vi "ReversedEngineering GetClassAttributes.vi"(1 "Path(CtrlRenum used if Path is empty)":path, 2 "CtlRefnum":refnum<vi>, 5 "error in (no error)":errorcluster) -> (12 "LibraryName":string, 15 "attributeInfo":T1[](array[typedef]), 19 "error out":errorcluster)   [LabVIEW 2020]
uses:
  <resource>/Framework/Providers/Open_GDS/UML/UmlEditor_class/UmlEditor.lvclass
  <resource>/Framework/Providers/Open_GDS/ClassProviders/Common/CommonVIs/CommonVIs_AttributeInfoType.ctl
  <resource>/Framework/Providers/Open_GDS/ClassProviders/Common/CommonVIs/CommonVIs_VisibilityType.ctl
  <resource>/Framework/Providers/Open_GDS/ClassProviders/Common/CommonVIs/CommonVIs_AttributeDataType.ctl
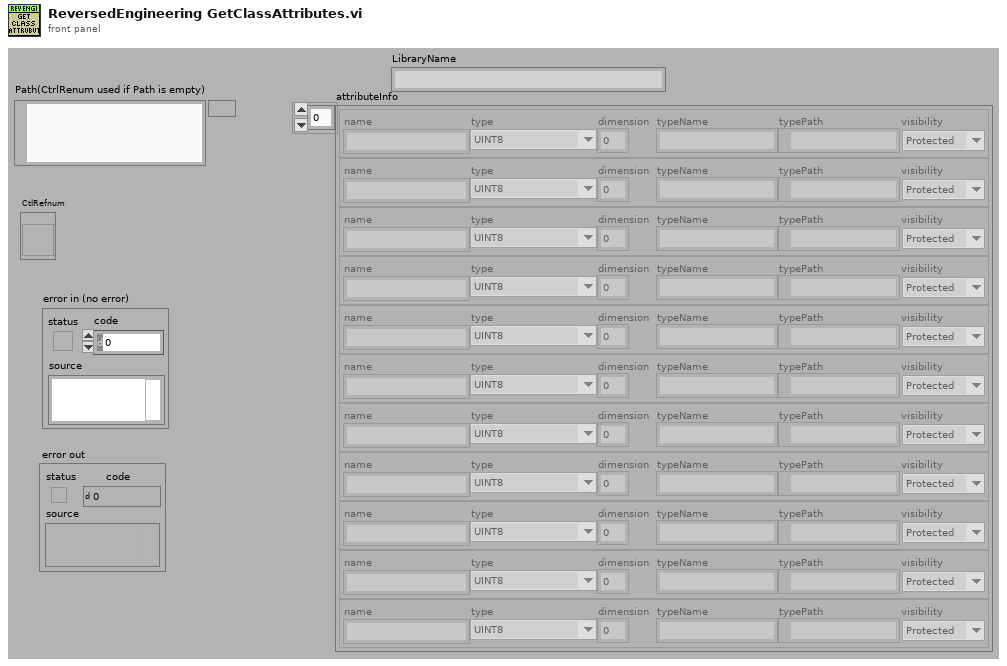
[diagram p1: front panel]
types:
  T1 = typedef "CommonVIs_AttributeInfoType.ctl" = cluster{"name":string, "type":T2, "dimension":i32, "typeName":string, "typePath":path, "visibility":T3}
  T2 = typedef "CommonVIs_AttributeDataType.ctl" = enum16{"UINT8", "INT8", "UINT16", "INT16", "UINT32", "INT32", "UINT64", "INT64", "SGL", "DBL", "EXT", "CSG", "CDB", "CXT", "TimeStamp", "STRING", "PATH", "BOOL", "ENUM", "RefNum", "VIRefNum", "LabVIEW Class", "Cluster", "Variant", "TypeDef", "Waveform", "LabVIEW Object", "Other", "void", "Set", "Map"}
  T3 = typedef "CommonVIs_VisibilityType.ctl" = enum16{"Public", "Private", "Protected"}
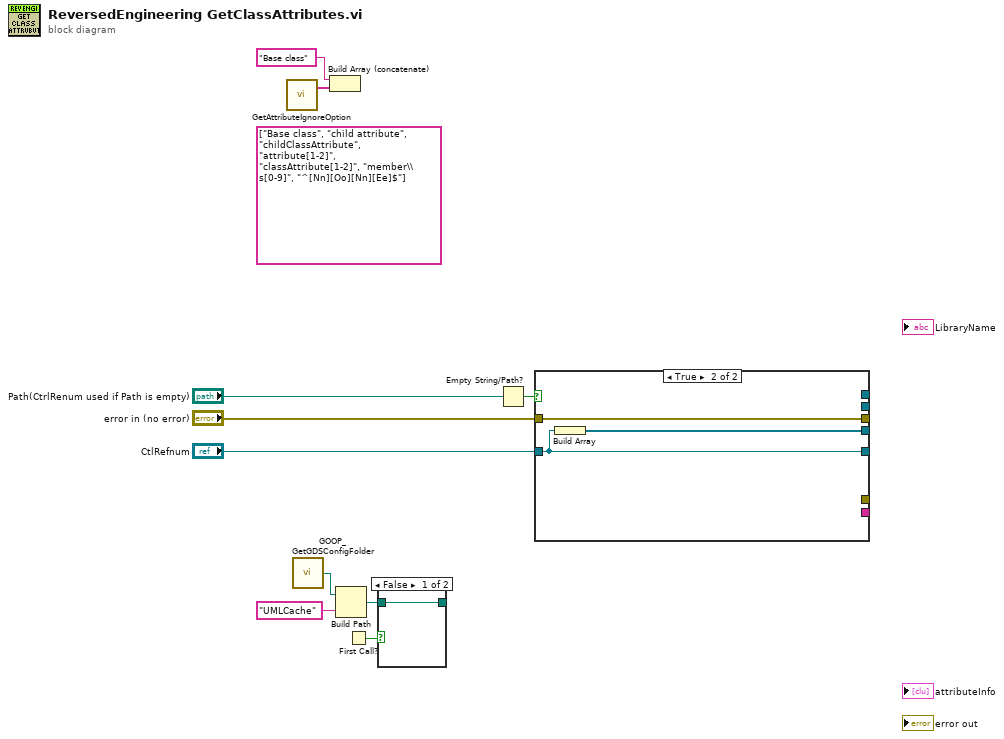
[diagram p0: block diagram]
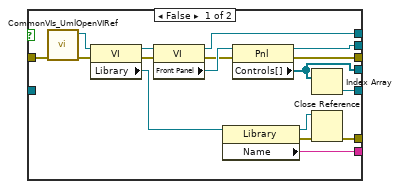
[diagram p2: hidden frame]
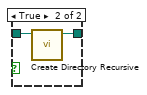
[diagram p3: hidden frame]
diagram:
  (unwired) string[] ["Base class", "child attribute", "childClassAttribute", "attribute[1-2]", "classAttribute[1-2]", "member\\s[0-9]", "^[Nn][Oo][Nn][Ee]$"]
  n1 = call <resource>:"GetAttributeIgnoreOption.vi"() -> ("Attr"=w8:string[])  [unwired: 1 in, 18 out]
  n2 = call <resource>:"GOOP_GetGDSConfigFolder.vi"() -> ("GDSFolderPath"=w4:path)
  n3 = Build Array (concatenate)("Base class", w8) -> ()  [unwired: 1 out]
  n4 = Build Path(base path=w4, name or relative path="UMLCache") -> (appended path=w7:path)
  n5 = First Call?() -> (First Call?: T/F=w6:bool)
  n6 = case shown="False" w6 {
    tunnel: w7 -> [w11 w13]
    tunnel: [w11 w12] -> _
    frame False {
    }
    frame True {
      n7 = call <vilib>:"Create Directory Recursive.vi"("directory"=w13) -> ("directory copy"=w12:path)  [unwired: 4 in, 2 out]
    }
  }
  n8 = Empty String/Path?(string/path="Path(CtrlRenum used if Path is empty)") -> (empty?=w3:bool)
  n9 = case shown="True" w3 {
    tunnel: [w27 w32] -> _
    tunnel: [w25 _] -> _
    tunnel: [w24 _] -> _
    tunnel: [w23 w31] -> _
    tunnel: [w22 w33] -> _
    tunnel: "error in (no error)" -> [w17 w33]
    tunnel: "CtlRefnum" -> [_ w32]
    tunnel: [w20 _] -> _
    tunnel: [w14 _] -> _
    frame False {
      n10 = call <resource>:"CommonVIs_UmlOpenVIRef.vi"("error in"=w17) -> ("error out"=w19:errorcluster, "vi reference"=w18:refnum<vi>)  [unwired: 3 in, 6 out]
      n11 = property class="VI"(reference=w18, error in=w19) -> (reference out=w30:refnum<vi>, error out=w29:errorcluster, "Library"=w21:refnum<vi>)
      n12 = property class="VI"(reference=w30, error in=w29) -> (reference out=w25:refnum<vi>, error out=w26:errorcluster, "Front Panel"=w28:refnum<vi>)
      n13 = property class="Library"(reference=w21) -> (reference out=w16:refnum<vi>, error out=w15:errorcluster, "Name"=w20:string)  [unwired: 1 in]
      n14 = property class="Pnl"(reference=w28, error in=w26) -> (reference out=w24:refnum<vi>, error out=w22:errorcluster, "Controls[]"=w23:refnum<vi>[])
      n15 = Index Array(array=w23) -> (element=w27:refnum<vi>)  [unwired: 1 in]
      n16 = Close Reference(reference=w16, error in (no error)=w15) -> (error out=w14:errorcluster)
    }
    frame True {
      n17 = Build Array(w32) -> (w31:refnum<vi>[])
    }
  }
